vi "Read Facility Code.vi"(8 "error in (no error)":errorcluster, 11 "abs_EventLog in":refnum<class "abs_EventLog.lvclass">) -> (0 "error out":errorcluster, 2 "Facility Code":T1=enum."user", 3 "abs_EventLog out":refnum<class "abs_EventLog.lvclass">)   [LabVIEW 2021, in "abs_EventLog.lvclass"]
uses:
  abs_EventLog.lvclass
  Support/Facility Code.ctl
  abs_EventLog.lvclass/abs_EventLog.ctl
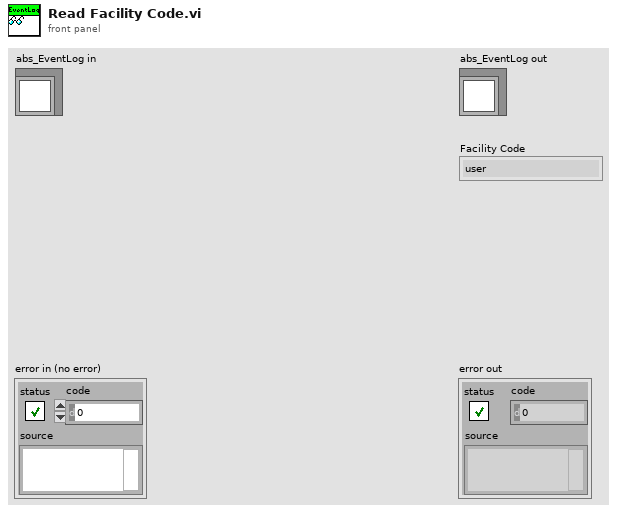
[diagram p1: front panel]
types:
  T1 = typedef "abs_EventLog.lvclass/Facility Code.ctl" = enum16{"kernel", "user", "mail", "system daemons", "security/authorization", "syslogd", "line printer", "network news", "uucp", "clock daemon", "security/authorization (alternate)", "FTP daemon", "NTP subsystem", "log audit", "log alert", "clock daemon (alternate)", "local use 0", "local use 1", "local use 2", "local use 3", "local use 4", "local use 5", "local use 6", "local use 7"}
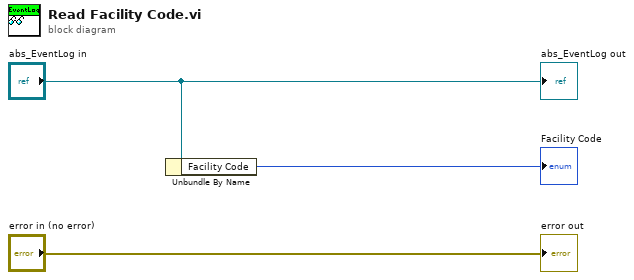
[diagram p0: block diagram]
diagram:
  n1 = Unbundle By Name("abs_EventLog in") -> ("Facility Code"=→"Facility Code":T1)
  "error out" <- "error in (no error)"
  "abs_EventLog out" <- "abs_EventLog in"
